vi "save images.vi"(8 "error in":errorcluster, 10 "path":string, 11 "image queue in":refnum<queue>) -> (0 "error out":errorcluster)   [LabVIEW 2025, in "Automotive Vision.lvclass"]
uses:
  Automotive Vision.lvclass
  image.ctl
  Automotive Vision.lvclass/Automotive Vision.ctl
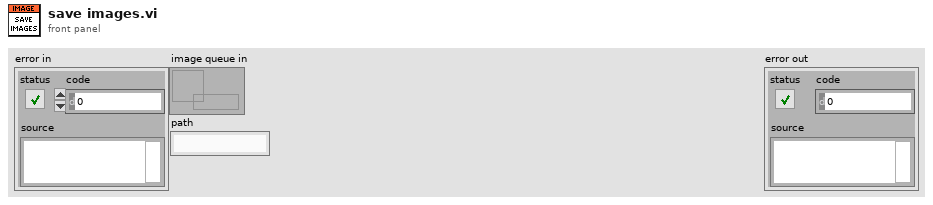
[diagram p1: front panel]
types:
  T1 = enum16{"open", "replace", "create", "open or create", "replace or create", "replace or create with confirmation"}
  T2 = typedef "Automotive Vision.lvclass/image.ctl" = cluster{"Frame ID":u32, "Data":u8[]}
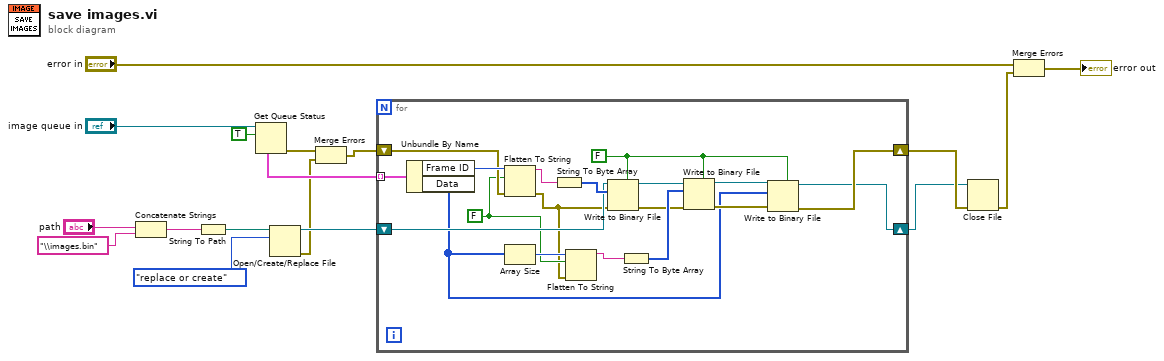
[diagram p0: block diagram]
diagram:
  n1 = Concatenate Strings("path", "\\images.bin" ("element")) -> (w3:string)
  n2 = String To Path(string=w3) -> (path=w2:path)
  n3 = Get Queue Status(queue="image queue in", return elements? (F)=TRUE) -> (error out=w8:errorcluster, elements=w15:T2[])  [unwired: 1 in, 6 out]
  n4 = Open/Create/Replace File(file path (use dialog)=w2, operation (0:open)=T1."replace or create") -> (refnum out=w14:refnum<file>, error out=w6:errorcluster)  [unwired: 4 in, 1 out]
  n5 = Merge Errors(w8, w6) -> (w7:errorcluster)
  n6 = for {
    tunnel: w15 -> [w36] mode=indexing
    shift-right: [w19] -> w13
    shift-left: w7 -> [w34]
    shift-right: [w18] -> w1
    shift-left: w14 -> [w31]
    w21 = FALSE ("prepend array or string size? (T)")
    w29 = FALSE
    n7 = Unbundle By Name(w36) -> ("Frame ID"=w35:u32, "Data"=w20:u8[])
    n8 = Flatten To String(anything=w35, prepend array or string size? (T)=w29, error in (no error)=w34) -> (data string=w33:string, error out=w27:errorcluster)  [unwired: 1 in, 1 out]
    n9 = Array Size(array=w20) -> (size(s)=w30:i32)
    n10 = String To Byte Array(string=w33) -> (unsigned byte array=w32:u8[])
    n11 = Flatten To String(anything=w30, prepend array or string size? (T)=w29, error in (no error)=w27) -> (data string=w28:string)  [unwired: 1 in, 2 out]
    n12 = Write to Binary File(file (use dialog)=w31, data=w32, error in=w27, 5:w21) -> (refnum out=w26:refnum<file>, error out=w24:errorcluster)  [unwired: 2 in, 1 out]
    n13 = String To Byte Array(string=w28) -> (unsigned byte array=w25:u8[])
    n14 = Write to Binary File(file (use dialog)=w26, data=w25, error in=w24, 5:w21) -> (refnum out=w23:refnum<file>, error out=w22:errorcluster)  [unwired: 2 in, 1 out]
    n15 = Write to Binary File(file (use dialog)=w23, data=w20, error in=w22, 5:w21) -> (refnum out=w18:refnum<file>, error out=w19:errorcluster)  [unwired: 2 in, 1 out]
  }
  n16 = Close File(refnum=w1, error in=w13) -> (error out=w11:errorcluster)  [unwired: 1 out]
  n17 = Merge Errors("error in", w11) -> (→"error out":errorcluster)
